vi "2014 Target Detection Gearheads.vi"(0 "Src Image":T3) -> (14 "Distances":T2(array[cluster]), 19 "Hot Target":bool)   [LabVIEW 2013]
uses:
  <vilib>/vision/Image Controls.llb/IMAQ Image.ctl
  TargetType.ctl
panel:
  in  "Std Devs":cluster{"Hue":dbl, "Sat":dbl, "Val":dbl}={"Hue"=4.0, "Sat"=6.0, "Val"=4.0}
  in  "Area Size Limit %":dbl=0.06 format="%#_13g"
  in  "Camera Type":enum16{"206", "1011", "1013"}(ring)=enum."1013"
  in  "Score Cutoff":dbl(slide)=54.248366013071895 scale=0.0..100.0
  in  "Color Components":T4={"Hue"={110.0, 142.0}, "Sat"={138.0, 255.0}, "Val"={139.0, 198.0}} {"Val" scale=0.0..255.0; "Sat" scale=0.0..255.0; "Hue" scale=0.0..255.0 scale format="%#_3g"}
  out "Image":T3(plugin-control)
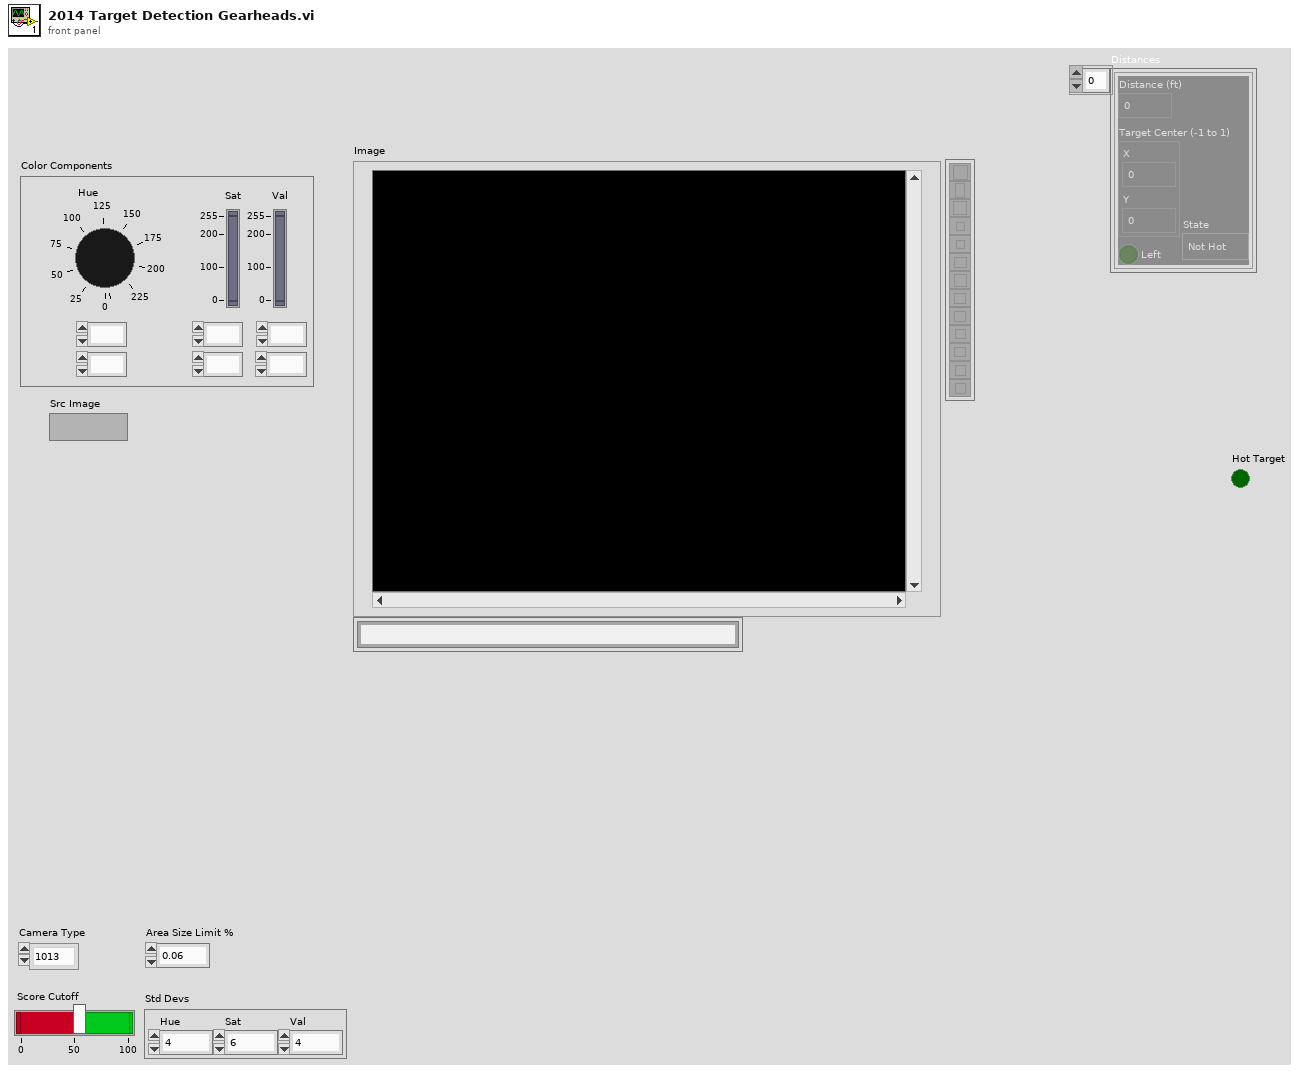
[diagram p1: front panel]
types:
  T1 = typedef "TargetType.ctl" = enum16{"Not Hot", "Hot"}
  T2 = cluster{"Distance (ft)":dbl, "Target Center (-1 to 1)":cluster{"X":dbl, "Y":dbl}, "Left":bool, "State":T1}[]
  T3 = typedef "IMAQ Image.ctl" = refnum<image>
  T4 = cluster{"Hue":cluster{dbl, dbl}, "Sat":cluster{dbl, dbl}, "Val":cluster{dbl, dbl}}
  T5 = cluster{cluster{dbl, dbl}, cluster{dbl, dbl}, cluster{dbl, dbl}}
  T6 = cluster{"Horizontal":bool, "Aspect Score":dbl, "Rect Score":dbl, cluster{"Left":dbl, "Top":dbl, "Right":dbl, "Bottom":dbl}, "Equiv H":dbl, "Equiv V":dbl}[]
  T7 = cluster{"Scores":cluster{"Total":dbl, "Left":dbl, "Right":dbl, "Ratio":dbl, "Vertical":dbl, "index":i32, "State":T1}, "Verticals":cluster{"Horizontal?":bool, "Aspect Score":dbl, "Rect Score":dbl, cluster{"Left":dbl, "Top":dbl, "Right":dbl, "Bottom":dbl}, "Equiv H":dbl, "Equiv V":dbl}, "Horizontals":cluster{"Horizontal?":bool, "Aspect Score":dbl, "Rect Score":dbl, cluster{"Left":dbl, "Top":dbl, "Right":dbl, "Bottom":dbl}, "Equiv H":dbl, "Equiv V":dbl}, "Validated":bool}[]
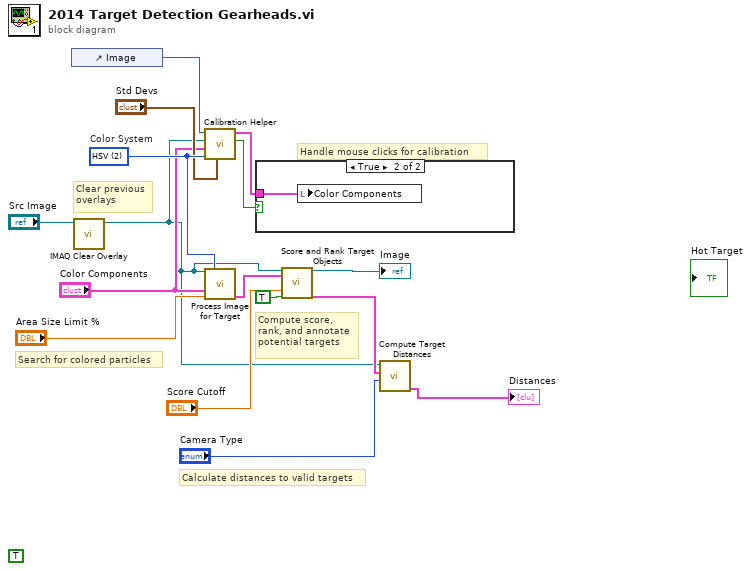
[diagram p0: block diagram]
diagram:
  w9 = u16 2 items=["RGB", "HSL", "HSV", "HSI"]  # Color System
  (unwired) TRUE
  # "Clear previous\noverlays"
  # "Calculate distances to valid targets"
  # "Search for colored particles"
  # "Handle mouse clicks for calibration"
  # "Compute score,\nrank, and annotate\npotential targets"
  n1 = control-ref of="Image"() -> (w10:refnum<vi>)
  n2 = call "IMAQ Clear Overlay"("Image"="Src Image") -> ("Image Out"=w1:T3)  [unwired: 9 in, 1 out]
  n3 = call "Calibration Helper.vi"("Std Devs"="Std Devs", "Color Mode"=w9, "Color Components"="Color Components", "Image"=w1, "Image Ctl Refnum"=w10) -> ("Changed"=w5:bool, "output color"=w7:T5)  [unwired: 5 in]
  n4 = call "Process Image for Target.vi"("Src Image"=w1, "Color Mode"=w9, "Color Components"="Color Components", "Area Cutoff %"="Area Size Limit %") -> ("Particles"=w13:T6)  [unwired: 9 in, 2 out]
  n5 = case shown="True" w5 {
    tunnel: w7 -> [_ w17]
    frame False {
    }
    frame True {
      n6 = local write "Color Components"(w17) -> ()
    }
  }
  n7 = call "Score and Rank Target Objects.vi"("Image in"=w1, "Particles"=w13, "Score Limit"="Score Cutoff", "Annotate"=TRUE) -> ("Annotated Image"=→"Image":T3, "Target Info"=w12:T7)  [unwired: 14 in]
  n8 = call "Compute Target Distances.vi"("Camera Type"="Camera Type", "Target Info"=w12, "Image in"=w1) -> ("Distances"=→"Distances":T2)  [unwired: 6 in, 2 out]
